vi "Verify Child Safety.vi"(0 "Lines":tag, 1 "GEA2 Reference In":refnum<k24>, 5 "Rate (Hz)":dbl=100.0 format="%0.2f", 7 "Samples":i32=1100, 9 "Cycle #":u8, 11 "Error In":errorcluster, 12 "MC Cycle Engine State":T1=enum."Start") -> (3 "GEA2 Reference Out":refnum<k24>, 4 "High Times (s)":dbl[][](array[numeric])=[[0.048, 19.932000000000002, 0.0], [0.256, 9.626, 10.098], [0.254, 9.628, 10.098], [0.256, 9.625, 10.099], [0.047, 19.933, 0.0], [0.253, 10.701, 9.026], [0.255, 10.699, 9.026], [0.048, 19.932000000000002, 0.0], [0.258, 8.014, 11.708], [0.256, 8.016, 11.708], [0.256, 8.016, 11.708], [0.048, 19.932000000000002, 0.0], [0.254, 7.527, 12.199], [0.047, 19.933, 0.0], [0.253, 6.848, 12.879]], 15 "Error Out":errorcluster)   [LabVIEW 2016, in "Centauro.lvlib"]
doc: "This VI reads multiple digital input lines and provides an array output of high/low times."
uses:
  Projects/Centauro.lvlib
  Q:/Common/DLLs/GEA3/GeaCommunication.dll
  Common/DLLs/GEA3/GeaCommunication.dll
  Valew Common/type defs/MC_Cycle_Engine_Request_State.ctl
  Common/LabVIEW GEA2 Toolkit/LabVIEW_GEA2_Toolkit.lvlibp/type defs/Source_Destination.ctl
  <vilib>/DAQmx/read.llb/DAQmx Read (Digital 1D Wfm NChan NSamp).vi
  <vilib>/DAQmx/create/channels.llb/DAQmx Create Channel (DI-Digital Input).vi
  <vilib>/DAQmx/configure/timing.llb/DAQmx Timing (Sample Clock).vi
  <vilib>/DAQmx/miscellaneous.llb/DAQmx Fill In Error Info.vi
  Common/LabVIEW GEA2 Toolkit/LabVIEW_GEA2_Toolkit.lvlibp
panel:
  out "Digital Waveform Graph":digitalwaveform[](graph)
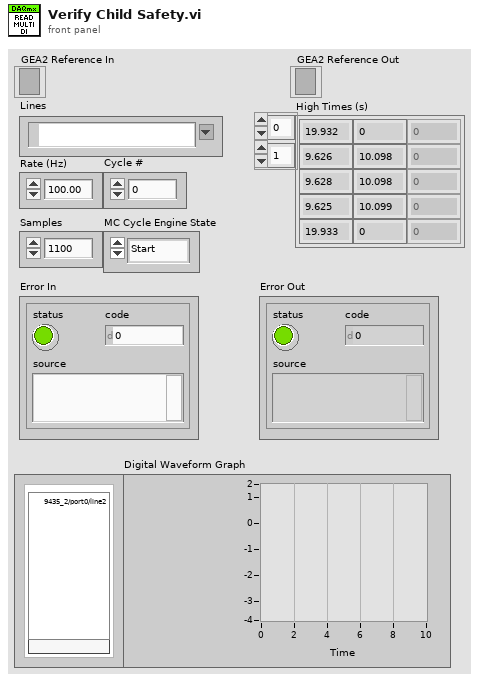
[diagram p1: front panel]
types:
  T1 = typedef "Centauro.lvlib/MC_Cycle_Engine_Request_State.ctl" = enum16{"Select", "Start", "Pause", "Resume", "Stop"}
  T2 = typedef "LabVIEW_GEA2_Toolkit.lvlibp/Source_Destination.ctl" = cluster{"Source":u8, "Destination":u8}
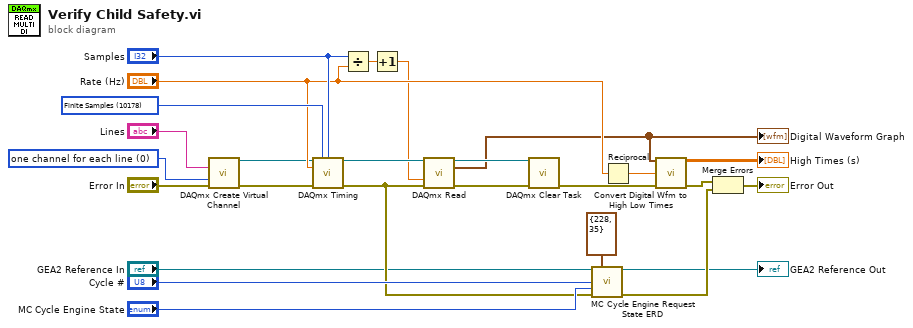
[diagram p0: block diagram]
diagram:
  w21 = 10178 items=["Finite Samples"=10178, "Continuous Samples"=10123, "Hardware Timed Single Point"=12522] ("sample mode")
  w26 = 0 items=["one channel for each line", "one channel for all lines"] ("line grouping")
  n1 = call-poly <vilib>:"DAQmx Create Virtual Channel.vi"("lines"="Lines", "line grouping"=w26, "error in"="Error In") -> ("task out"=w10:refnum<k21>, "error out"=w11:errorcluster)  [unwired: 11 in]
  n2 = call-poly <vilib>:"DAQmx Timing.vi"("task/channels in"=w10, "sample mode"=w21, "samples per channel"="Samples", "rate"="Rate (Hz)", "error in"=w11) -> ("task out"=w22:refnum<k21>, "error out"=w2:errorcluster)  [unwired: 9 in]
  n3 = Divide(x="Samples", y="Rate (Hz)") -> (x/y=w16:dbl)
  n4 = Increment(x=w16) -> (x+1=w15:dbl)
  n5 = call-poly <vilib>:"DAQmx Read.vi"("task/channels in"=w22, "timeout"=w15, "error in"=w2) -> ("task out"=w25:refnum<k21>, "data"=w13:digitalwaveform[], "error out"=w9:errorcluster)  [unwired: 10 in]
  "Digital Waveform Graph" <- w13
  n6 = call <vilib>:"DAQmx Clear Task.vi"("task in"=w25, "error in"=w9) -> ("error out"=w19:errorcluster)  [unwired: 13 in]
  n7 = call "MC Cycle Engine Request State ERD.vi"("GEA2 Reference In"="GEA2 Reference In", "GEA Inputs"=T2 {"Source"=228, "Destination"=35}, "Cycle #"="Cycle #", "MC Cycle Engine State"="MC Cycle Engine State", "Error In"=w2) -> ("GEA2 Reference Out"=→"GEA2 Reference Out":refnum<k24>, "Error Out"=w4:errorcluster)  [unwired: 9 in]
  n8 = Reciprocal(x="Rate (Hz)") -> (1/x=w20:dbl)
  n9 = call "Convert Digital Wfm to High Low Times.vi"("Digital Waveform In"=w13, "Dt"=w20, "Error In"=w19) -> ("HL Raw Output"=→"High Times (s)":dbl[][], "Error Out"=w6:errorcluster)  [unwired: 11 in]
  n10 = Merge Errors(w6, w4) -> (→"Error Out":errorcluster)
